vi "Read Configuration Parameters.vi"(8 "error in (no error)":errorcluster, 10 "refnum":T1, 11 "Example Configuration Dialog in":refnum<class "Server Config.lvclass">) -> (0 "error out":errorcluster, 2 "refnum out 2":T1, 3 "Example Configuration Dialog out":refnum<class "Server Config.lvclass">)   [LabVIEW 2026, in "Server Controller.lvlib" / "Server Config.lvclass"]
uses:
  Server Config.lvclass
  <vilib>/Utility/config.llb/Config Data RefNum.ctl
  Server Config.lvclass/Server Config.ctl
  framework/Msmt Configuration/Controller Configuration.lvclass
  <vilib>/Utility/config.llb/NI_LVConfig.lvlib
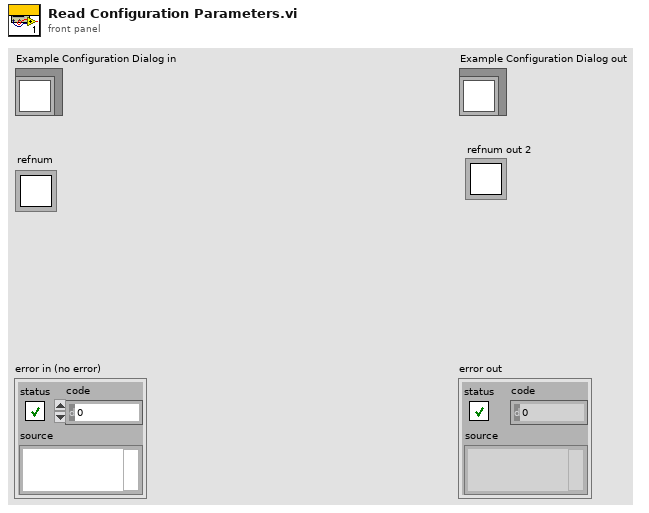
[diagram p1: front panel]
types:
  T1 = typedef "NI_LVConfig.lvlib/Config Data RefNum.ctl" = refnum<k1>
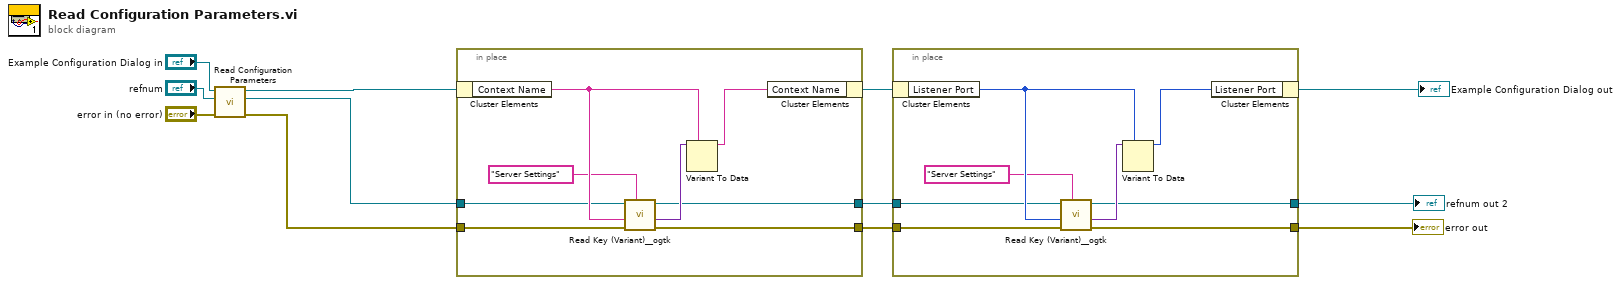
[diagram p0: block diagram]
diagram:
  n1 = call-parent "Read Configuration Parameters.vi"("error in (no error)"="error in (no error)", "refnum"="refnum", "Example Configuration Dialog in"="Example Configuration Dialog in") -> ("error out"=w7:errorcluster, "refnum out"=w8:T1, "Example Configuration Dialog out"=w9:refnum<class "Server Config.lvclass">)  [unwired: 6 in]
  n2 = in-place {
    in-place-border: w8 -> [w17]
    in-place-border: [w16] -> w6
    in-place-border: w7 -> [w15]
    in-place-border: [w14] -> w5
    n3 = in-place-cluster #1(w9) -> ("Context Name"=w20:string)
    n4 = call <userlib>:"Read Key (Variant)__ogtk.vi"("section"="Server Settings", "error in (no error)"=w15, "type"=w20, "refnum"=w17) -> ("error out"=w14:errorcluster, "key-value"=w19:variant, "refnum out"=w16:T1)  [unwired: 4 in, 1 out]
    n5 = Variant To Data(type=w20, Variant=w19) -> (data=w18:string)  [unwired: 1 in, 1 out]
    n6 = in-place-cluster #1("Context Name"=w18) -> (w4:refnum<class "Server Config.lvclass">)
  }
  n7 = in-place {
    in-place-border: w6 -> [w25]
    in-place-border: [w24] -> w2
    in-place-border: w5 -> [w23]
    in-place-border: [w22] -> w1
    n8 = in-place-cluster #2(w4) -> ("Listener Port"=w28:u16)
    n9 = call <userlib>:"Read Key (Variant)__ogtk.vi"("section"="Server Settings", "error in (no error)"=w23, "type"=w28, "refnum"=w25) -> ("error out"=w22:errorcluster, "key-value"=w27:variant, "refnum out"=w24:T1)  [unwired: 4 in, 1 out]
    n10 = Variant To Data(type=w28, Variant=w27) -> (data=w26:u16)  [unwired: 1 in, 1 out]
    n11 = in-place-cluster #2("Listener Port"=w26) -> (→"Example Configuration Dialog out":refnum<class "Server Config.lvclass">)
  }
  "error out" <- w1
  "refnum out 2" <- w2
